vi "OpenPython.vi"() -> (3 "session out":refnum<k35>)   [LabVIEW 2018]
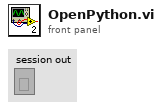
[diagram p1: front panel]
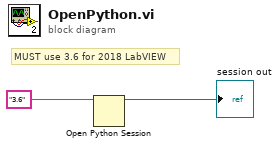
[diagram p0: block diagram]
diagram:
  # "MUST use 3.6 for 2018 LabVIEW"
  n1 = Open Python Session(python version="3.6" ("Python version")) -> (session out=→"session out":refnum<k35>)  [unwired: 2 in, 1 out]
